vi "ReduceSize.generated.vi"(11 "buffer.in":u64[](array[numeric])=[0, 0, 0, 0, 0, 0, 0, 0, 0]) -> (3 "OrderBook.Command":T1)   [LabVIEW 2020]
doc: "Cboe PITCH Reduce Size (0x25 long, 0x26 short) -> orderbook.command: type ReduceSize, orderId, canceled.qty, nanoseconds (time offset), Edit flag. Same structure as AddOrder.vi."
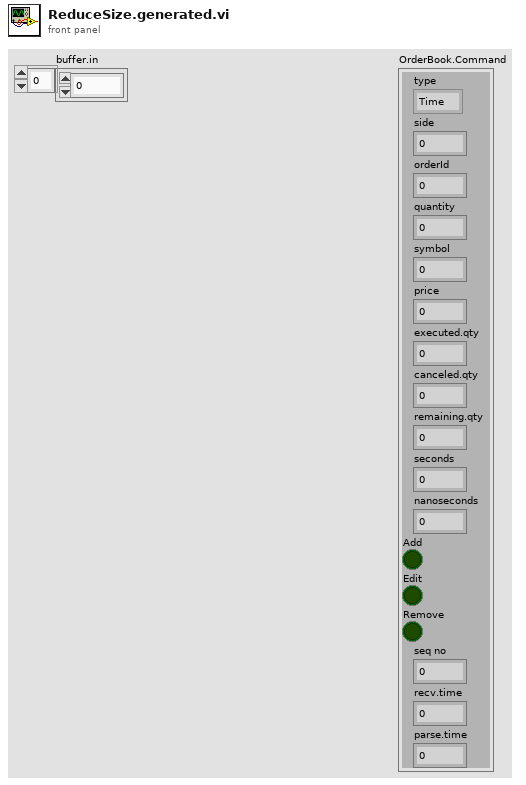
[diagram p1: front panel]
types:
  T1 = cluster{"type":enum8{"Time", "AddOrder", "OrderExecuted", "OrderExecutedAtPrice", "ReduceSize", "ModifyOrder", "DeleteOrder", "Get.Everything", "Get.All.Orders", "Get.Top"}, "side":u8, "orderId ":u64, "quantity":u32, "symbol":u64, "price":u64, "executed.qty":u32, "canceled.qty":u32, "remaining.qty":u32, "seconds":u64, "nanoseconds":u64, "Add":bool, "Edit":bool, "Remove":bool, "seq no":u32, "recv.time":u64, "parse.time":u64}
  T2 = enum8{"Time", "AddOrder", "OrderExecuted", "OrderExecutedAtPrice", "ReduceSize", "ModifyOrder", "DeleteOrder", "Get.Everything", "Get.All.Orders", "Get.Top"}
  T3 = cluster{"type":enum8{"Time", "AddOrder", "OrderExecuted", "OrderExecutedAtPrice", "ReduceSize", "ModifyOrder", "DeleteOrder", "Get.Everything", "Get.All.Orders", "Get.Top"}, "side":u8, "orderId ":u64, "quantity":u32, "symbol":u64, "price":u64, "executed.qty":u32, u32, "remaining.qty":u32, "seconds":u64, "nanoseconds":u64, "Add":bool, "Edit":bool, "Remove":bool, "seq no":u32, "recv.time":u64, "parse.time":u64}
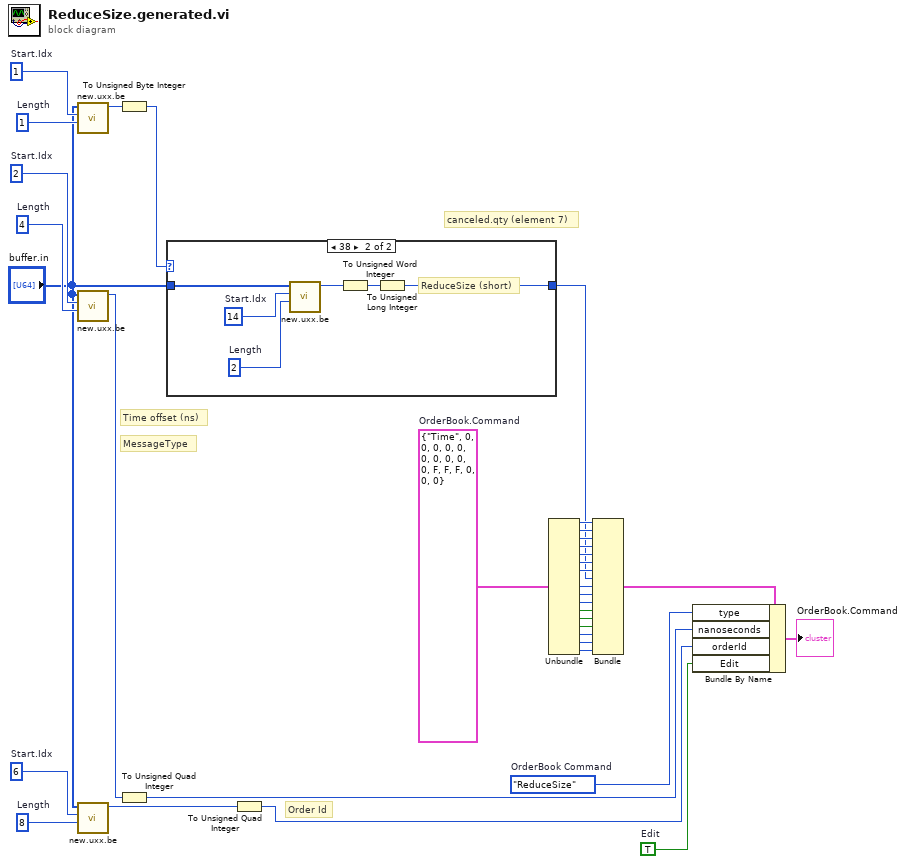
[diagram p0: block diagram]
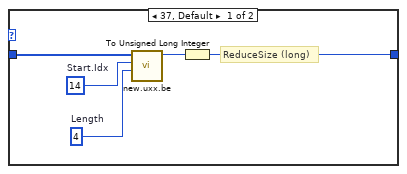
[diagram p2: hidden frame]
diagram:
  w30 = u8 8  # Length
  w31 = u8 6  # Start.Idx
  w32 = u8 4  # Length
  w33 = u8 2  # Start.Idx
  w34 = u8 1  # Length
  w35 = u8 1  # Start.Idx
  w3 = TRUE  # Edit
  w24 = T1 {"type"=enum."Time", "side"=0, "orderId "=0, "quantity"=0, "symbol"=0, "price"=0, "executed.qty"=0, "canceled.qty"=0, "remaining.qty"=0, "seconds"=0, "nanoseconds"=0, "Add"=FALSE, "Edit"=FALSE, "Remove"=FALSE, "seq no"=0, "recv.time"=0, "parse.time"=0}  # OrderBook.Command
  w6 = T2."ReduceSize"  # OrderBook Command
  # "canceled.qty (element 7)"
  # "Order Id"
  # "Time offset (ns)"
  # "MessageType"
  n1 = call "new.uxx.be.vi"("buffer (U64)"="buffer.in", "Start.Idx"=w35, "Length"=w34) -> ("Out.Value U64"=w29:u64)  [unwired: 7 in]
  n2 = call "new.uxx.be.vi"("buffer (U64)"="buffer.in", "Start.Idx"=w33, "Length"=w32) -> ("Out.Value U64"=w28:u64)  [unwired: 7 in]
  n3 = call "new.uxx.be.vi"("buffer (U64)"="buffer.in", "Start.Idx"=w31, "Length"=w30) -> ("Out.Value U64"=w27:u64)  [unwired: 7 in]
  n4 = To Unsigned Byte Integer(number=w29) -> (unsigned 8bit integer=w25:u8)
  n5 = To Unsigned Quad Integer(1:w28) -> (0:w5:u64)
  n6 = case shown="38" w25 {
    tunnel: "buffer.in" -> [w40 w46]
    tunnel: [w36 w41] -> w16
    frame 37, Default {
      w38 = u8 4  # Length
      w39 = u8 14  # Start.Idx
      # "ReduceSize (long)"
      n7 = call "new.uxx.be.vi"("buffer (U64)"=w40, "Start.Idx"=w39, "Length"=w38) -> ("Out.Value U64"=w37:u64)  [unwired: 7 in]
      n8 = To Unsigned Long Integer(number=w37) -> (unsigned 32bit integer=w36:u32)
    }
    frame 38 {
      w44 = u8 2  # Length
      w45 = u8 14  # Start.Idx
      # "ReduceSize (short)"
      n9 = call "new.uxx.be.vi"("buffer (U64)"=w46, "Start.Idx"=w45, "Length"=w44) -> ("Out.Value U64"=w43:u64)  [unwired: 7 in]
      n10 = To Unsigned Word Integer(number=w43) -> (unsigned 16bit integer=w42:u16)
      n11 = To Unsigned Long Integer(number=w42) -> (unsigned 32bit integer=w41:u32)
    }
  }
  n12 = To Unsigned Quad Integer(1:w27) -> (0:w4:u64)
  n13 = Unbundle(w24) -> ("type"=w23:T2, "side"=w22:u8, "orderId"=w21:u64, "quantity"=w20:u32, "symbol"=w19:u64, "price"=w18:u64, "executed.qty"=w17:u32, "remaining.qty"=w15:u32, "seconds"=w14:u64, "nanoseconds"=w13:u64, "Add"=w12:bool, "Edit"=w11:bool, "Remove"=w10:bool, "seq no"=w9:u32, "recv.time"=w8:u64, "parse.time"=w7:u64)  [unwired: 1 out]
  n14 = Bundle("type"=w23, "side"=w22, "orderId"=w21, "quantity"=w20, "symbol"=w19, "price"=w18, "executed.qty"=w17, w16, "remaining.qty"=w15, "seconds"=w14, "nanoseconds"=w13, "Add"=w12, "Edit"=w11, "Remove"=w10, "seq no"=w9, "recv.time"=w8, "parse.time"=w7) -> (w2:T3)  [unwired: 1 in]
  n15 = Bundle By Name(cluster=w2, "type"=w6, "nanoseconds"=w5, "orderId"=w4, "Edit"=w3) -> (→"OrderBook.Command":T3)
